vi "Configure Connector.vi"(8 "error in (no error)":errorcluster, 9 "Connector (RF1COM)":i32(ring)=1 items=["RF1COM"=1, "RF2COM"=2, "RF3COM"=3, "RF4COM"=4, "RF5COM"=5, "RF6COM"=6, "IF1IN"=7, "IF2IN"=8, "IF3IN"=9], 10 "Instance (1)":T1=1, 11 "VISA resource name":refnum<visa-resource-name>) -> (0 "error out":errorcluster, 3 "VISA resource name out":refnum<visa-resource-name>)   [LabVIEW 2015, in "Rohde&Schwarz CMXP NR FR2 Measurement.lvlib"]
doc: "Selects the input connector for the measured signal.\n\nAttribute:\nRSCMXPNRFR2M_ATTR_CONNECTOR\n\nRemote-control command:\nROUTe:NRMMw:MEAS<i>:SPATh"
uses:
  <instrlib>/Rohde&Schwarz CMXP NR FR2 Measurement/Rohde&Schwarz CMXP NR FR2 Measurement.lvlib
  <instrlib>/Rohde&Schwarz CMXP NR FR2 Measurement/Private/_Instance.ctl
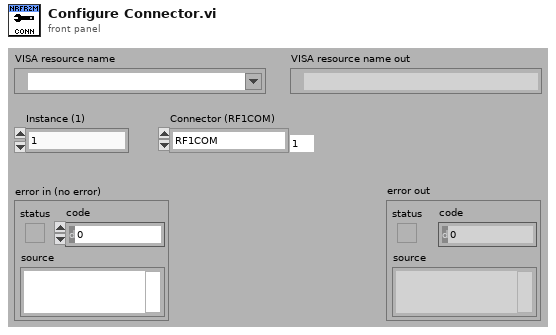
[diagram p1: front panel]
types:
  T1 = typedef "Rohde&Schwarz CMXP NR FR2 Measurement.lvlib/_Instance.ctl" = i32
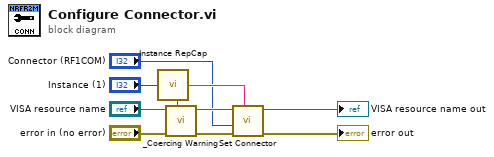
[diagram p0: block diagram]
diagram:
  n1 = call <instrlib>:"Instance RepCap.vi"("Instance In"="Instance (1)") -> ("In Range?"=w6:bool, "RepCap Identifier Out"=w3:string)  [unwired: 1 in]
  n2 = call <instrlib>:"_Coercing Warning.vi"("In Range?"=w6, "error in (no error)"="error in (no error)", "VISA resource name"="VISA resource name") -> ("error out"=w4:errorcluster, "VISA resource name out"=w5:refnum<visa-resource-name>)  [unwired: 7 in]
  n3 = call "Set Connector"("Repeated Capabilities"=w3, "error in (no error)"=w4, "Connector (1 - RF1COM)"="Connector (RF1COM)", "instrument handle"=w5) -> ("error out"=→"error out":errorcluster, "instrument handle out"=→"VISA resource name out":refnum<visa-resource-name>)  [unwired: 6 in]
